vi "Ic readout.vi"() -> ()   [LabVIEW 2021]
uses:
  <vilib>/LabVIEW Targets/FPGA/cRIO/shared/nicrio_ModuleControls/nicrio_cRIO-9775_TriggerSlope.ctl
  <vilib>/LabVIEW Targets/FPGA/cRIO/shared/nicrio_ModuleControls/nicrio_BasicConversionTime.ctl
  <vilib>/LabVIEW Targets/FPGA/cRIO/shared/nicrio_ModuleControls/nicrio_cRIO-9775_RecordDataRates4ChansRing.ctl
  <vilib>/rvi/Emulation/niFpgaGetClockAttributes.vi
  <vilib>/rvi/Emulation/niFpgaSctlEmulationGetInTimedLoop.vi
  <vilib>/rvi/Emulation/niFpgaEmulationReportErrorSimple.vi
  <vilib>/rvi/Emulation/niFpgaProcessEmulError.vi
  <vilib>/rvi/eio/common/nirviEmuTemplateMethod_errors.vi
  <vilib>/rvi/Emulation/niFpgaCriticalErrorInLSC.vi
  <vilib>/rvi/eio/common/nirviEmuTemplatePropertySet_errors.vi
  <vilib>/rvi/interface/RandomDataEmulation/niFpgaRandomDataHandleErrors.vi
  <vilib>/eio/EIOMethodNode/EIOMethodNode.xnode
  <vilib>/eio/EIONode/EIONode.xnode
  <vilib>/eio/EIOPropertyNode/EIOPropertyNode.xnode
  <vilib>/rvi/DataTransferAndStorage/Container/XNode/niFpgaContainer.xnode
  <vilib>/rvi/interface/RandomDataEmulation/nirviRandomDataFpgaReadWriteTemplate.vi
  <vilib>/rvi/eio/common/nirviEmuTemplatePropertyGet_errors.vi
  <vilib>/rvi/eio/common/nirviEmuTemplatePropertyGet_noerrors.vi
  <vilib>/rvi/eio/common/nirviEmuTemplatePropertySet_noerrors.vi
panel:
  in  "Gate wait time us":u32=100 caption="Count(uSec)"
  in  "Ic Cut off or curve":bool
  in  "Timeout":i32=-1
  in  "Record Samples":u32=25
  in  "Record PreTrigger Samples":u32=1
  in  "Record Data Rate":T1=1 items=["20.000 MS/s (NI 9775)"=1, "10.00 MS/s (NI 9775)"=2, "6.667 MS/s (NI 9775)"=3, "5.000 MS/s (NI 9775)"=4, "2.500 MS/s (NI 9775)"=8, "1.667 MS/s (NI 9775)"=12, "1.250 MS/s (NI 9775)"=16, "1.000 MS/s (NI 9775)"=20, "833.333 KS/s (NI 9775)"=24, "714.286 KS/s (NI 9775)"=28, "625.000 KS/s (NI 9775)"=32, "555.556 KS/s (NI 9775)"=36, "500.000 KS/s (NI 9775)"=40, "454.545 KS/s (NI 9775)"=44, "416.667 KS/s (NI 9775)"=48, "384.615 KS/s (NI 9775)"=52, "357.143 KS/s (NI 9775)"=56, "333.333 KS/s (NI 9775)"=60, "312.500 KS/s (NI 9775)"=64, "294.118 KS/s (NI 9775)"=68, "277.778 KS/s (NI 9775)"=72, "263.158 KS/s (NI 9775)"=76, "250.000 KS/s (NI 9775)"=80, "238.095 KS/s (NI 9775)"=84, "227.273 KS/s (NI 9775)"=88, "217.391 KS/s (NI 9775)"=92, "208.333 KS/s (NI 9775)"=96, "200.000 KS/s (NI 9775)"=100, "192.308 KS/s (NI 9775)"=104, "185.185 KS/s (NI 9775)"=108, "178.571 KS/s (NI 9775)"=112, "172.414 KS/s (NI 9775)"=116, "166.667 KS/s (NI 9775)"=120, "161.290 KS/s (NI 9775)"=124, "156.250 KS/s (NI 9775)"=128, "151.515 KS/s (NI 9775)"=132, "147.059 KS/s (NI 9775)"=136, "142.857 KS/s (NI 9775)"=140, "138.889 KS/s (NI 9775)"=144, "135.135 KS/s (NI 9775)"=148, "131.579 KS/s (NI 9775)"=152, "128.205 KS/s (NI 9775)"=156, "125.000 KS/s (NI 9775)"=160, "121.951 KS/s (NI 9775)"=164, "119.048 KS/s (NI 9775)"=168, "116.279 KS/s (NI 9775)"=172, "113.636 KS/s (NI 9775)"=176, "111.111 KS/s (NI 9775)"=180, "108.696 KS/s (NI 9775)"=184, "106.383 KS/s (NI 9775)"=188, "104.167 KS/s (NI 9775)"=192, "102.041 KS/s (NI 9775)"=196, "100.000 KS/s (NI 9775)"=200, "50.000 KS/s (NI 9775)"=400, "33.333 KS/s (NI 9775)"=600, "25.000 KS/s (NI 9775)"=800, "20.000 KS/s (NI 9775)"=1000, "16.667 KS/s (NI 9775)"=1200, "14.286 KS/s (NI 9775)"=1400, "12.500 KS/s (NI 9775)"=1600, "11.111 KS/s (NI 9775)"=1800, "10.000 KS/s (NI 9775)"=2000, "9.091 KS/s (NI 9775)"=2200, "8.333 KS/s (NI 9775)"=2400, "7.692 KS/s (NI 9775)"=2600, "7.143 KS/s (NI 9775)"=2800, "6.667 KS/s (NI 9775)"=3000, "6.250 KS/s (NI 9775)"=3200, "5.882 KS/s (NI 9775)"=3400, "5.556 KS/s (NI 9775)"=3600, "5.000 KS/s (NI 9775)"=4000, "4.762 KS/s (NI 9775)"=4200, "4.545 KS/s (NI 9775)"=4400, "4.348 KS/s (NI 9775)"=4600, "4.167 KS/s (NI 9775)"=4800, "4.000 KS/s (NI 9775)"=5000, "3.846 KS/s (NI 9775)"=5200, "3.571 KS/s (NI 9775)"=5600, "3.333 KS/s (NI 9775)"=6000, "3.125 KS/s (NI 9775)"=6400, "2.941 KS/s (NI 9775)"=6800, "2.778 KS/s (NI 9775)"=7200, "2.632 KS/s (NI 9775)"=7600, "2.500 KS/s (NI 9775)"=8000, "2.381 KS/s (NI 9775)"=8400, "2.273 KS/s (NI 9775)"=8800, "2.174 KS/s (NI 9775)"=9200, "2.083 KS/s (NI 9775)"=9600, "2.000 KS/s (NI 9775)"=10000, "1.923 KS/s (NI 9775)"=10400, "1.852 KS/s (NI 9775)"=10800, "1.786 KS/s (NI 9775)"=11200, "1.724 KS/s (NI 9775)"=11600, "1.667 KS/s (NI 9775)"=12000, "1.613 KS/s (NI 9775)"=12400, "1.563 KS/s (NI 9775)"=12800, "1.515 KS/s (NI 9775)"=13200, "1.471 KS/s (NI 9775)"=13600, "1.429 KS/s (NI 9775)"=14000, "1.389 KS/s (NI 9775)"=14400, "1.351 KS/s (NI 9775)"=14800, "1.316 KS/s (NI 9775)"=15200, "1.282 KS/s (NI 9775)"=15600, "1.250 KS/s (NI 9775)"=16000, "1.220 KS/s (NI 9775)"=16400, "1.190 KS/s (NI 9775)"=16800, "1.163 KS/s (NI 9775)"=17200, "1.136 KS/s (NI 9775)"=17600, "1.111 KS/s (NI 9775)"=18000, "1.087 KS/s (NI 9775)"=18400, "1.064 KS/s (NI 9775)"=18800, "1.042 KS/s (NI 9775)"=19200, "1.020 KS/s (NI 9775)"=19600, "1.000 KS/s (NI 9775)"=20000, "0.980 KS/s (NI 9775)"=20400, "0.962 KS/s (NI 9775)"=20800, "0.943 KS/s (NI 9775)"=21200, "0.926 KS/s (NI 9775)"=21600, "0.909 KS/s (NI 9775)"=22000, "0.893 KS/s (NI 9775)"=22400, "0.877 KS/s (NI 9775)"=22800, "0.862 KS/s (NI 9775)"=23200, "0.847 KS/s (NI 9775)"=23600, "0.833 KS/s (NI 9775)"=24000, "0.820 KS/s (NI 9775)"=24400, "0.806 KS/s (NI 9775)"=24800, "0.794 KS/s (NI 9775)"=25200, "0.781 KS/s (NI 9775)"=25600, "0.694 KS/s (NI 9775)"=28800, "0.625 KS/s (NI 9775)"=32000, "0.568 KS/s (NI 9775)"=35200, "0.521 KS/s (NI 9775)"=38400, "0.446 KS/s (NI 9775)"=44800, "0.391 KS/s (NI 9775)"=51200, "0.347 KS/s (NI 9775)"=57600, "0.313 KS/s (NI 9775)"=64000]
  in  "Timing Mode":T2
  in  "Records Num":i32=1
  in  "AI Trigger Configuration":T4={"Trigger Slope"=enum."Positive", "Trigger Level"=1.199951171875, "Hystesis Value"=1.10009765625, "AI Channel"=0}
  out "error out":errorcluster
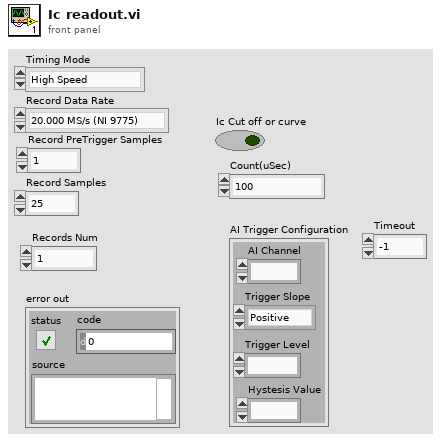
[diagram p1: front panel]
types:
  T1 = typedef "nicrio_cRIO-9775_RecordDataRates4ChansRing.ctl" = u16
  T2 = typedef "nicrio_BasicConversionTime.ctl" = enum8{"High Speed", "High Resolution"}
  T3 = typedef "nicrio_cRIO-9775_TriggerSlope.ctl" = enum8{"Positive", "Negative"}
  T4 = cluster{"Trigger Slope":T3, "Trigger Level":fxp<+/-,17,5>, "Hystesis Value":fxp<+,16,4>, "AI Channel":u8}
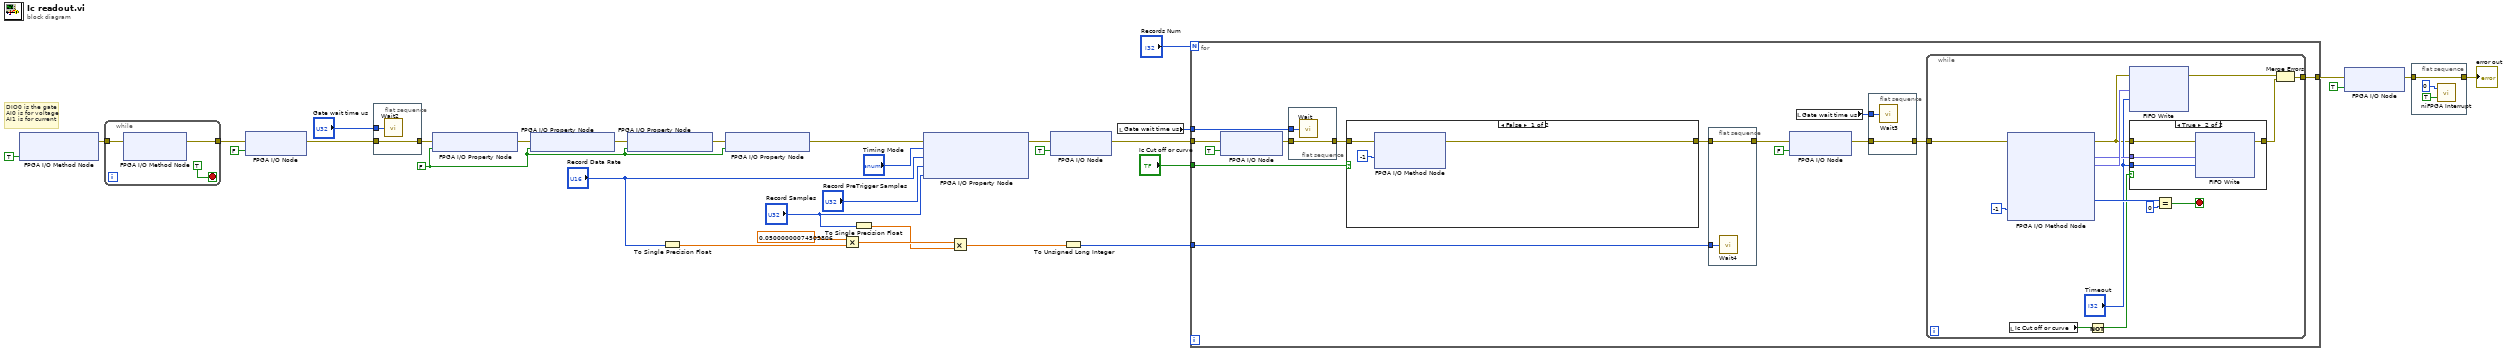
[diagram p0: block diagram]
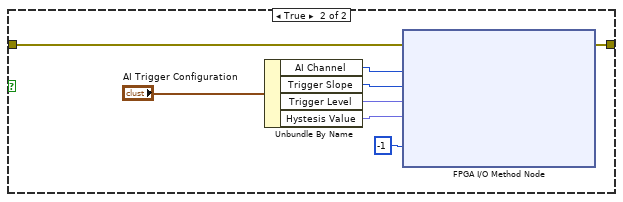
[diagram p2: hidden frame]
diagram:
  w22 = FALSE ("Enable Low Pass Filter")
  # "DIO0 is the gate\nAI0 is for voltage\nAI1 is for current"
  n1 = xnode "FPGA I/O Method Node"("Enable"=TRUE) -> ("error out"=w28:errorcluster)  [unwired: 2 in, 1 out]
  n2 = while {
    tunnel: w28 -> [w35]
    tunnel: [w34] -> w27
    stop <- TRUE stop-if-true
    n3 = xnode "FPGA I/O Method Node"("error in"=w35) -> ("error out"=w34:errorcluster)  [unwired: 1 in, 2 out]
  }
  n4 = xnode "FPGA I/O Node"("error in"=w27, "Mod2/DIO0"=FALSE) -> ("error out"=w15:errorcluster)  [unwired: 1 in, 1 out]
  n5 = flat-sequence {
    tunnel: w15 -> [w37]
    tunnel: [w37] -> w14
    tunnel: "Gate wait time us" -> [w36]
    frame #0 {
      n6 = call "Wait2"("Count(uSec)"=w36) -> ()  [unwired: 1 out]
    }
  }
  n7 = xnode "FPGA I/O Property Node"("error in"=w14, "Enable Analog Filter"=w22) -> ("error out"=w26:errorcluster)  [unwired: 1 in, 1 out]
  n8 = xnode "FPGA I/O Property Node"("error in"=w26, "Enable Analog Filter"=w22) -> ("error out"=w24:errorcluster)  [unwired: 1 in, 1 out]
  n9 = xnode "FPGA I/O Property Node"("error in"=w24, "Enable Analog Filter"=w22) -> ("error out"=w23:errorcluster)  [unwired: 1 in, 1 out]
  n10 = To Single Precision Float(number="Record Data Rate") -> (single precision float=w6:sgl)
  n11 = xnode "FPGA I/O Property Node"("error in"=w23, "Enable Analog Filter"=w22) -> ("error out"=w21:errorcluster)  [unwired: 1 in, 1 out]
  n12 = Multiply(x=sgl 0.05, y=w6) -> (x*y=w5:sgl)
  n13 = To Single Precision Float(number="Record Samples") -> (single precision float=w3:sgl)
  n14 = xnode "FPGA I/O Property Node"("error in"=w21, "Timing Mode"="Timing Mode", "Record Data Rate"="Record Data Rate", "Record PreTrigger Samples"="Record PreTrigger Samples", "Record Samples"="Record Samples") -> ("error out"=w20:errorcluster)  [unwired: 1 in, 1 out]
  n15 = Multiply(x=w5, y=w3) -> (x*y=w2:sgl)
  n16 = xnode "FPGA I/O Node"("error in"=w20, "Mod1/Start"=TRUE) -> ("error out"=w25:errorcluster)  [unwired: 1 in, 1 out]
  n17 = To Unsigned Long Integer(number=w2) -> (unsigned 32bit integer=w1:u32)
  n18 = local read "Gate wait time us"() -> (w11:u32)
  n19 = for {
    N: "Records Num" -> [_]
    tunnel: w25 -> [w51]
    tunnel: "Ic Cut off or curve" -> [w48]
    tunnel: [w47] -> w12
    tunnel: w11 -> [w46]
    tunnel: w1 -> [w38]
    n20 = xnode "FPGA I/O Node"("error in"=w51, "Mod2/DIO0"=TRUE) -> ("error out"=w45:errorcluster)  [unwired: 1 in, 1 out]
    n21 = flat-sequence {
      tunnel: w46 -> [w57]
      tunnel: w45 -> [w56]
      tunnel: [w56] -> w44
      frame #0 {
        n22 = call "Wait"("Count(uSec)"=w57) -> ()  [unwired: 1 out]
      }
    }
    n23 = case shown="False" w48 {
      tunnel: w44 -> [w59 w68]
      tunnel: [w58 w62] -> w40
      frame False {
        n24 = xnode "FPGA I/O Method Node"("error in"=w59, "Timeout (Ticks)"=-1) -> ("error out"=w58:errorcluster)  [unwired: 1 in, 2 out]
      }
      frame True {
        n25 = Unbundle By Name("AI Trigger Configuration") -> ("AI Channel"=w67:u8, "Trigger Slope"=w66:T3, "Trigger Level"=w65:fxp<+/-,17,5>, "Hystesis Value"=w64:fxp<+,16,4>)
        n26 = xnode "FPGA I/O Method Node"("error in"=w68, "AI Channel"=w67, "Trigger Slope"=w66, "Trigger Level"=w65, "Hysteresis Value"=w64, "Timeout (Ticks)"=-1) -> ("error out"=w62:errorcluster)  [unwired: 1 in, 3 out]
      }
    }
    n27 = flat-sequence {
      tunnel: w40 -> [w53]
      tunnel: [w53] -> w39
      tunnel: w38 -> [w52]
      frame #0 {
        n28 = call "Wait4"("Count(uSec)"=w52) -> ()  [unwired: 1 out]
      }
    }
    n29 = xnode "FPGA I/O Node"("error in"=w39, "Mod2/DIO0"=FALSE) -> ("error out"=w43:errorcluster)  [unwired: 1 in, 1 out]
    n30 = local read "Gate wait time us"() -> (w42:u32)
    n31 = flat-sequence {
      tunnel: w42 -> [w55]
      tunnel: w43 -> [w54]
      tunnel: [w54] -> w41
      frame #0 {
        n32 = call "Wait3"("Count(uSec)"=w55) -> ()  [unwired: 1 out]
      }
    }
    n33 = while {
      tunnel: w41 -> [w82]
      tunnel: [w71] -> w47
      stop <- w78 stop-if-true
      n34 = xnode "FPGA I/O Method Node"("error in"=w82, "Timeout (Ticks)"=-1) -> ("error out"=w74:errorcluster, "AI0"=w76:fxp<+/-,17,5>, "AI1"=w77:fxp<+/-,17,5>, "Elements Remaining"=w80:u32)  [unwired: 1 in, 5 out]
      n35 = local read "Ic Cut off or curve"() -> (w70:bool)
      n36 = Not(x=w70) -> (.not. x?=w69:bool)
      n37 = xnode ("FIFO Write")("Element"=w77, "Timeout"="Timeout", "error in (no error)"=w74) -> ("error out"=w73:errorcluster)  [unwired: 1 in, 2 out]
      n38 = case shown="True" w69 {
        tunnel: w76 -> [_ w87]
        tunnel: "Timeout" -> [_ w86]
        tunnel: w74 -> [w83 w85]
        tunnel: [w83 w84] -> w72
        frame False {
        }
        frame True {
          n39 = xnode ("FIFO Write")("Element"=w87, "Timeout"=w86, "error in (no error)"=w85) -> ("error out"=w84:errorcluster)  [unwired: 1 in, 2 out]
        }
      }
      n40 = Equal?(x=w80, y=u32 0) -> (x = y?=w78:bool)
      n41 = Merge Errors(w73, w72) -> (w71:errorcluster)
    }
  }
  n42 = xnode "FPGA I/O Node"("error in"=w12, "Mod1/Stop"=TRUE) -> ("error out"=w10:errorcluster)  [unwired: 1 in, 1 out]
  n43 = flat-sequence {
    tunnel: w10 -> [w90]
    tunnel: [w90] -> w9
    frame #0 {
      n44 = call <vilib>:"niFPGA Interrupt.vi"("Wait Until Cleared (F)"=TRUE, "IRQ Number (0)"=u8 0) -> ()  [unwired: 1 in]
    }
  }
  "error out" <- w9
